vi "CompterRotationsDAQ.vi"(8 "Bouton Stop":bool, 9 "Énum":enum16{"lire", "commencer", "arreter"}(ring)=enum."commencer", 10 "pin":i32, 11 "daq":u32) -> (2 "Compteur":i32, 3 "AtHome":bool)   [LabVIEW 2020]
uses:
  <userlib>/cDaq/cDaq.lvlib
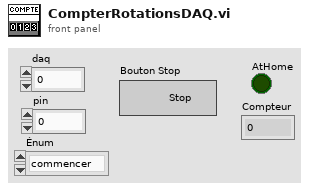
[diagram p1: front panel]
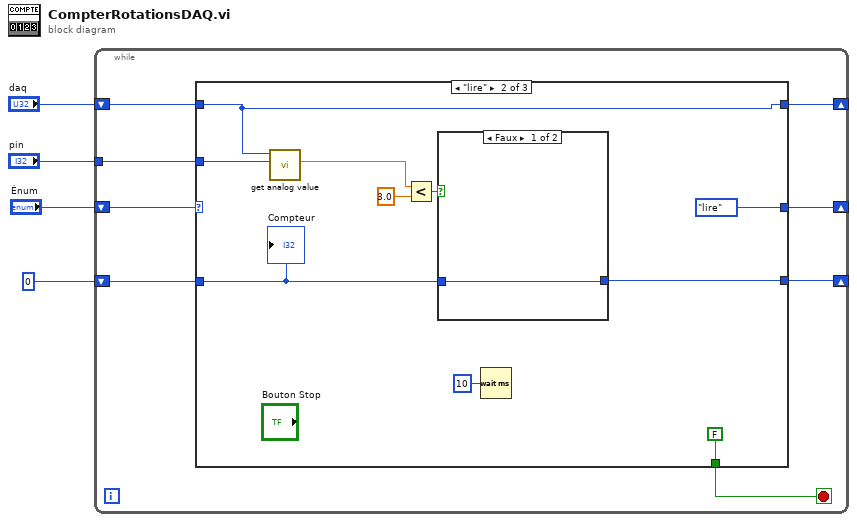
[diagram p0: block diagram]
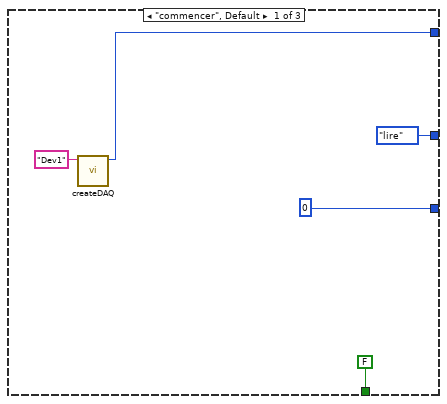
[diagram p2: hidden frame]
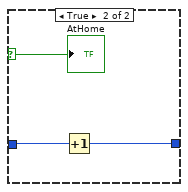
[diagram p3: hidden frame]
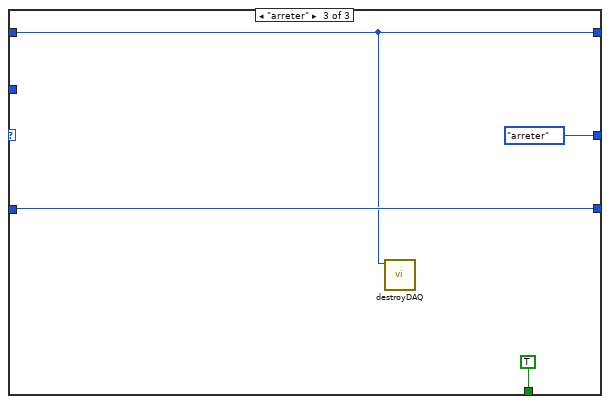
[diagram p4: hidden frame]
diagram:
  n1 = while {
    shift-right: [w10] -> _
    shift-left: 0 -> [w11]
    shift-right: [w6] -> _
    shift-left: "Énum" -> [w7]
    tunnel: "pin" -> [w8]
    shift-right: [w5] -> _
    shift-left: "daq" -> [w9]
    stop <- w12 stop-if-true
    n2 = case shown="\"lire\"" w7 {
      tunnel: [FALSE FALSE TRUE] -> w12
      tunnel: w11 -> [_ w25 w35]
      tunnel: [0 w24 w35] -> w10
      tunnel: w9 -> [_ w19 w33]
      tunnel: w8 -> [_ w20 _]
      tunnel: [enum16{"lire", "commencer", "arreter"}."lire" ("Énum") enum16{"lire", "commencer", "arreter"}."lire" ("Énum") enum16{"lire", "commencer", "arreter"}."arreter" ("Énum")] -> w6
      tunnel: [w14 w19 w33] -> w5
      frame "commencer", Default {
        n3 = call "createDAQ.vi"("device"="Dev1") -> ("function return"=w14:u32)  [unwired: 9 in]
      }
      frame "lire" {
        n4 = call <userlib>:"get analog value .vi"("pin"=w20, "daq"=w19) -> ("function return"=w27:dbl)  [unwired: 8 in, 1 out]
        n5 = Less?(x=w27, y=3.0) -> (x < y?=w23:bool)
        n6 = case shown="Faux" w23 {
          selector: w23 -> [_ w29]
          tunnel: w25 -> [w28 w31]
          tunnel: [w28 w30] -> w24
          frame False {
          }
          frame True {
            n7 = Increment(x=w31) -> (x+1=w30:i32)
            "AtHome" <- w29
          }
        }
        n8 = Wait (ms)(milliseconds to wait=u32 10 ("attente (ms)")) -> ()  [unwired: 1 out]
        "Compteur" <- w25
      }
      frame "arreter" {
        n9 = call "destroyDAQ.vi"("handle"=w33) -> ()  [unwired: 10 in, 1 out]
      }
    }
  }
